vi "Validate Status.vi"(0 "Error Msg[]":string[](array[string]), 5 "Error[]":errorcluster[](array[cluster]), 11 "error in (no error)":errorcluster) -> (4 "Status":string[](array[string]), 15 "error out":errorcluster)   [LabVIEW 2021, in "Packager Helpers.lvlib"]
uses:
  Packager Helpers.lvlib
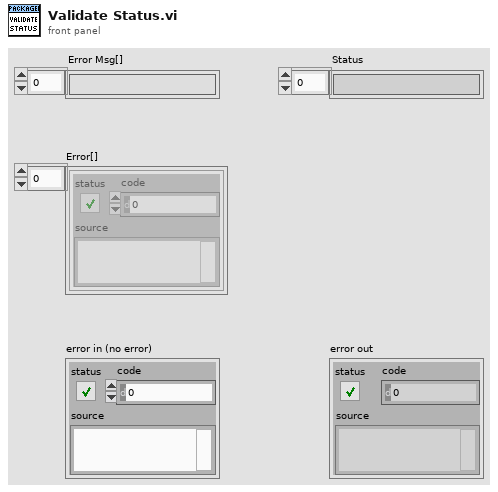
[diagram p1: front panel]
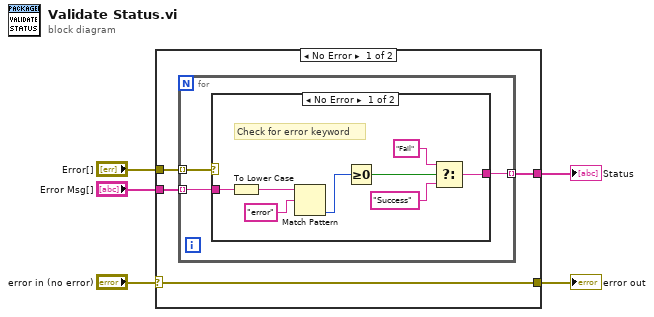
[diagram p0: block diagram]
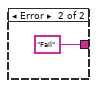
[diagram p2: hidden frame]
diagram:
  n1 = case shown="No Error" "error in (no error)" {
    selector: "error in (no error)" -> [w6 w22]
    tunnel: "Error[]" -> [w9 _]
    tunnel: "Error Msg[]" -> [w8 _]
    tunnel: [w7 _] -> w5
    tunnel: [w6 w22] -> w3
    frame No Error {
      n2 = for {
        tunnel: w9 -> [w12] mode=indexing
        tunnel: w8 -> [w11] mode=indexing
        tunnel: [w10] -> w7 mode=indexing
        n3 = case shown="No Error" w12 {
          tunnel: w11 -> [w20 _]
          tunnel: [w13 "Fail" ("regular expression")] -> w10
          frame No Error {
            # "Check for error keyword"
            n4 = To Lower Case(string=w20) -> (all lower case string=w19:string)
            n5 = Match Pattern(string=w19, regular expression="error") -> (offset past match=w17:i32)  [unwired: 1 in, 3 out]
            n6 = Greater Or Equal To 0?(x=w17) -> (x >= 0?=w16:bool)
            n7 = Select(t="Fail" ("regular expression"), s=w16, f="Success" ("regular expression")) -> (s? t:f=w13:string)
          }
          frame Error {
          }
        }
      }
    }
    frame Error {
    }
  }
  "error out" <- w3
  "Status" <- w5
